vi "Vision Example 4.vi"() -> ()   [LabVIEW 2014]
uses:
  <vilib>/userdefined/High Color/IMAQdx.ctl
  <vilib>/vision/driver/NI_Vision_Acquisition_Software.lvlib
panel:
  out "FindLaser Out":T1(plugin-control)
  in  "stop":bool
  out "Running":bool
  out "error out":errorcluster
  out "Live Input":T1(plugin-control)
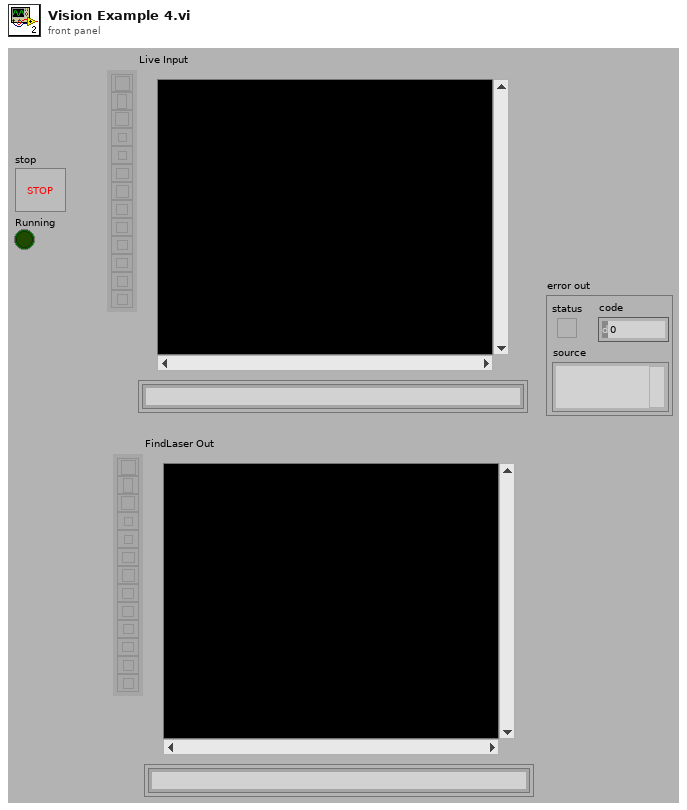
[diagram p1: front panel]
types:
  T1 = typedef "IMAQ Image.ctl" = refnum<image>
  T2 = typedef "Image Type" = u32
  T3 = typedef "IMAQdx.ctl" = refnum<k21>
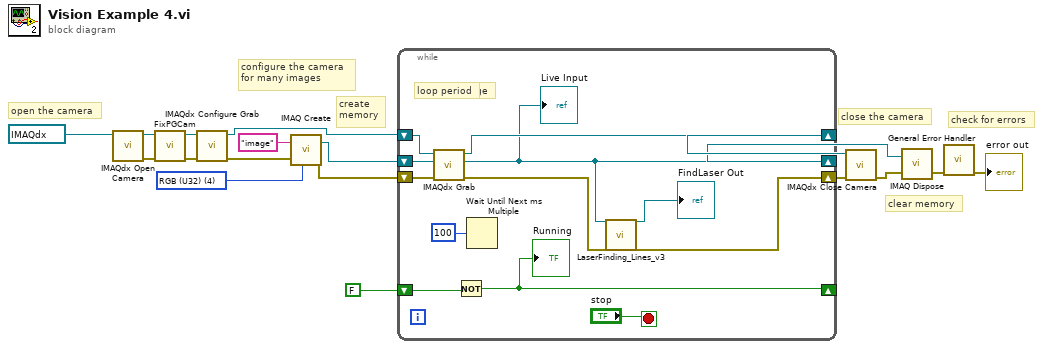
[diagram p0: block diagram]
diagram:
  w16 = T2 4 items=["Grayscale (U8)", "Grayscale (I16)", "Grayscale (SGL)", "Complex (CSG)", "RGB (U32)", "HSL (U32)", "RGB (U64)", "Grayscale (U16)"] ("Image Type")
  # "check for errors"
  # "clear memory"
  # "close the camera"
  # "create\nmemory"
  # "configure the camera\nfor many images"
  # "open the camera"
  n1 = call <vilib>:"IMAQdx Open Camera.vi"("Session In"=T3 "cam1") -> ("error out"=w2:errorcluster, "Session Out"=w1:T3)  [unwired: 2 in, 7 out]
  n2 = call "FixPGCam.vi"("error in"=w2, "Session In"=w1) -> ("error out"=w4:errorcluster, "IMAQdx Session Out"=w3:T3)  [unwired: 8 in]
  n3 = call <vilib>:"IMAQdx Configure Grab.vi"("error in"=w4, "Session In"=w3) -> ("error out"=w12:errorcluster, "Session Out"=w14:T3)  [unwired: 8 out]
  n4 = call "IMAQ Create"("Image Name"="image", "Image Type"=w16, "error in (no error)"=w12) -> ("New Image"=w13:T1, "error out"=w15:errorcluster)  [unwired: 1 in, 1 out]
  n5 = while {
    shift-right: [w26] -> w11
    shift-left: w14 -> [w29]
    shift-right: [w22] -> w8
    shift-left: w13 -> [w28]
    shift-right: [w19] -> w10
    shift-left: w15 -> [w27]
    shift-right: [w24] -> _
    shift-left: FALSE -> [w25]
    stop <- "stop" stop-if-true
    # "get one image"
    # "loop period"
    n6 = call <vilib>:"IMAQdx Grab.vi"("error in"=w27, "Image In"=w28, "Session In"=w29) -> ("error out"=w20:errorcluster, "Image Out"=w22:T1, "Session Out"=w26:T3)  [unwired: 1 in, 5 out]
    "Live Input" <- w22
    n7 = Not(x=w25) -> (.not. x?=w24:bool)
    "Running" <- w24
    n8 = Wait Until Next ms Multiple(millisecond multiple=u32 100 ("milliseconds to wait")) -> ()  [unwired: 1 out]
    n9 = call "LaserFinding_Lines_v3.vi"("Image In"=w22, "error in"=w20) -> ("Image Out"=→"FindLaser Out":T1, "error out"=w19:errorcluster)  [unwired: 22 in, 2 out]
  }
  n10 = call <vilib>:"IMAQdx Close Camera.vi"("error in"=w10, "Session In"=w11) -> ("error out"=w9:errorcluster)  [unwired: 9 out]
  n11 = call "IMAQ Dispose"("Image"=w8, "error in (no error)"=w9) -> ("error out"=w7:errorcluster)  [unwired: 1 in, 3 out]
  n12 = call <vilib>:"General Error Handler.vi"("error in (no error)"=w7) -> ("error out"=→"error out":errorcluster)  [unwired: 2 in, 12 out]
